vi "log_message.vi"(8 "error in (no error)":errorcluster, 9 "message":string, 11 "Logger in":refnum<class "WebSocket Logger.lvclass">) -> (0 "error out":errorcluster, 3 "Logger out":refnum<class "WebSocket Logger.lvclass">)   [LabVIEW 2019, in "WebSocket Server Toolkit.lvlib" / "WebSocket Logger.lvclass"]
uses:
  WebSocket Logger.lvclass
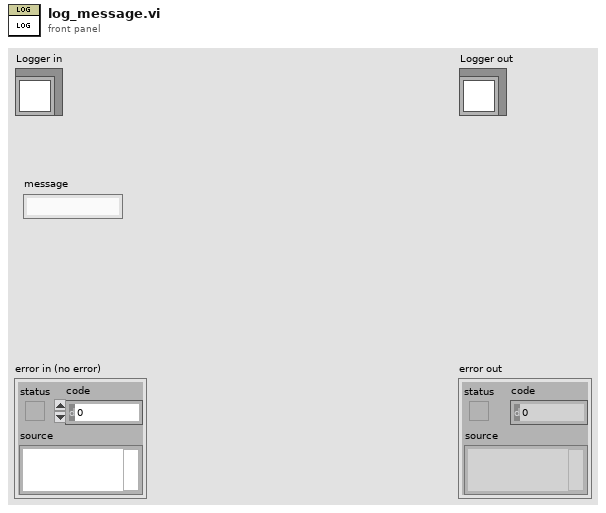
[diagram p1: front panel]
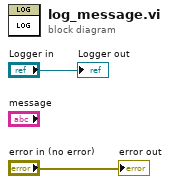
[diagram p0: block diagram]
diagram:
  "error out" <- "error in (no error)"
  "Logger out" <- "Logger in"
